vi "Destroy Stage Controller.vi"(8 "error in (no error)":errorcluster, 11 "XY Stage Controller in":refnum<class "XY Stage Controller.lvclass">) -> (0 "error out":errorcluster, 3 "XY Stage Controller out":refnum<class "XY Stage Controller.lvclass">)   [LabVIEW 2022 SP3, in "XY Stage Controller.lvclass"]
uses:
  XY Stage Controller.lvclass
  Process Framework/Interlock Q Class/Interlock Q Class.lvclass
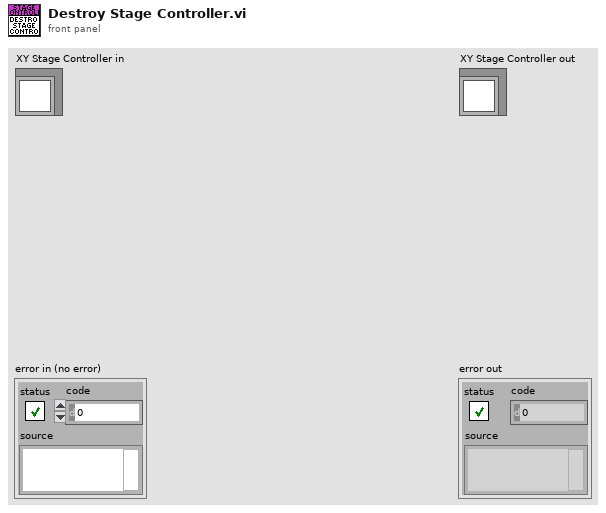
[diagram p1: front panel]
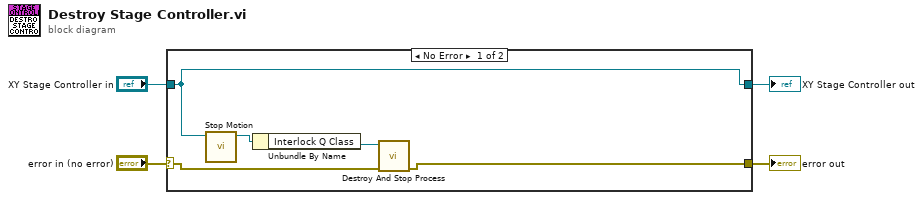
[diagram p0: block diagram]
diagram:
  n1 = case shown="No Error" "error in (no error)" {
    selector: "error in (no error)" -> [w7 w11]
    tunnel: [w6 w11] -> w3
    tunnel: [w5 w10] -> w1
    tunnel: "XY Stage Controller in" -> [w5 w10]
    frame No Error {
      n2 = call-dynamic "Stop Motion.vi"("2-Axis Stage in"=w5) -> ("2-Axis Stage out"=w9:refnum<class "XY Stage Controller.lvclass">)  [unwired: 9 in, 1 out]
      n3 = Unbundle By Name(w9) -> ("Interlock Q Class"=w8:refnum<class "Interlock Q Class.lvclass">)
      n4 = call-dynamic "Destroy And Stop Process.vi"("error in (no error)"=w7, "Interlock Q Class in"=w8) -> ("error out"=w6:errorcluster)  [unwired: 8 in, 1 out]
    }
    frame Error {
    }
  }
  "error out" <- w3
  "XY Stage Controller out" <- w1
